vi "NI9252_AnalogInputWaveforms_v2.vi"() -> ()   [LabVIEW 2025]
uses:
  <vilib>/DAQmx/read.llb/DAQmx Read (Analog 1D Wfm NChan NSamp).vi
  <vilib>/DAQmx/configure/timing.llb/DAQmx Timing (Sample Clock).vi
  <vilib>/DAQmx/miscellaneous.llb/DAQmx Fill In Error Info.vi
panel:
  out "error out":errorcluster
  out "AI6 - Angle Sensor":dynamicdata(graph)
  out "AI5 - Potentiometer Sensor":dynamicdata(graph)
  out "AI4 - Differential Pressure":dynamicdata(graph)
  out "AI3 - Chamber Pressure":dynamicdata(graph)
  out "AI1 - Flow Meter Pressure":dynamicdata(graph)
  out "AI2 - Inlet Pressure":dynamicdata(graph)
  out "AI0 - Supply Pressure":dynamicdata(graph)
  in  "stop":bool
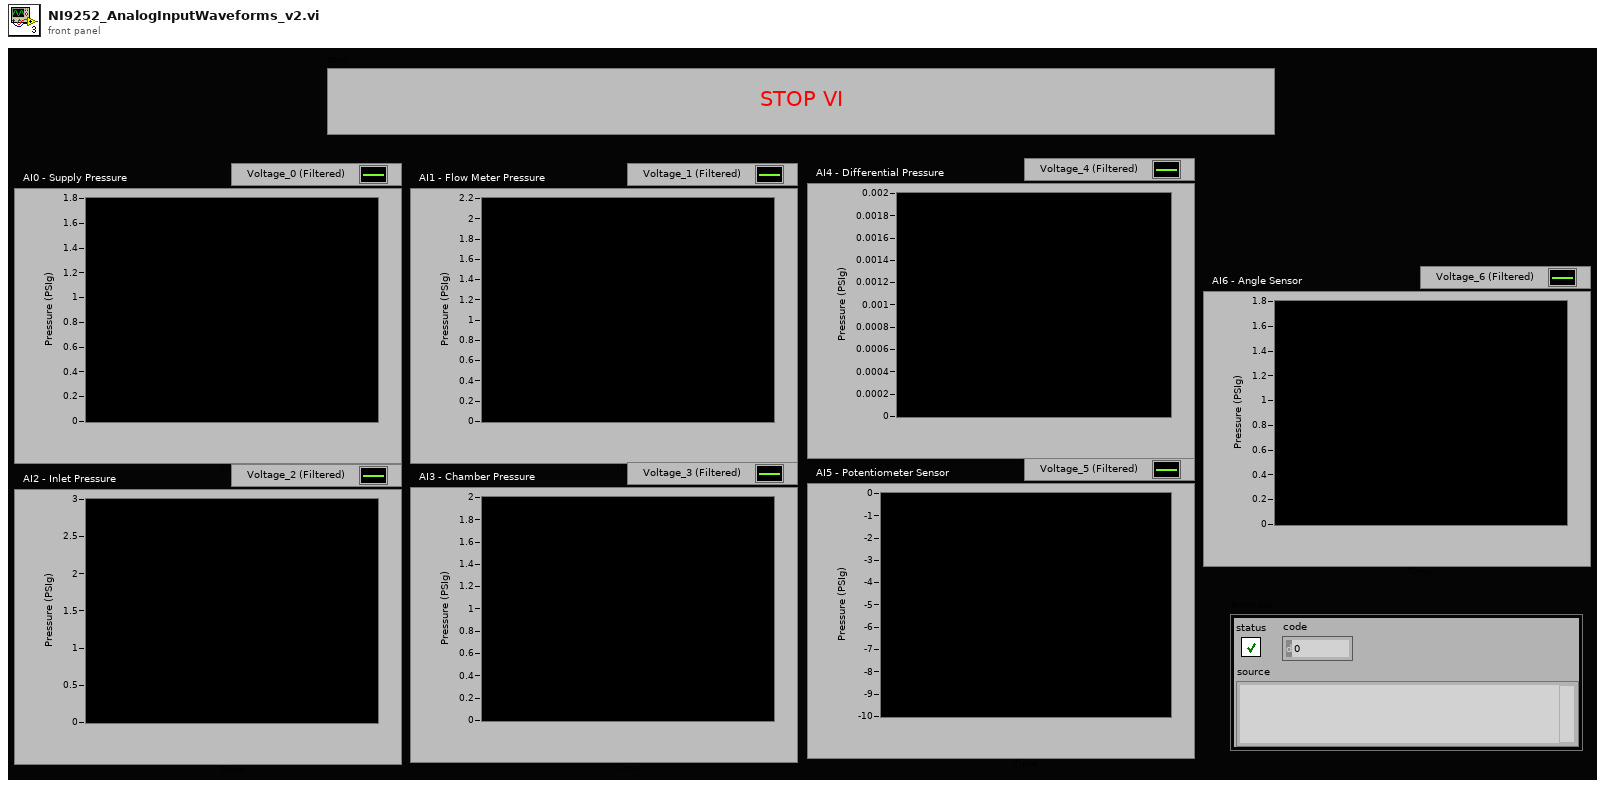
[diagram p1: front panel]
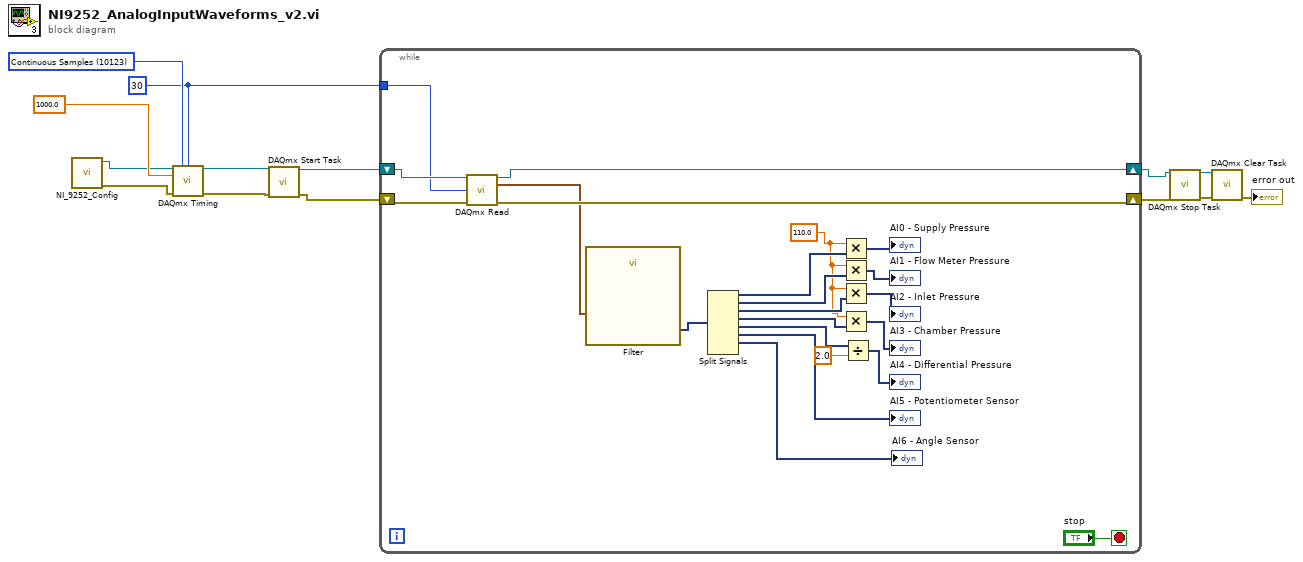
[diagram p0: block diagram]
diagram:
  w6 = 30 ("samples per channel")
  w7 = 10123 items=["Finite Samples"=10178, "Continuous Samples"=10123, "Hardware Timed Single Point"=12522] ("sample mode")
  n1 = call "NI_9252_Config.vi"() -> ("error out"=w12:errorcluster, "task out"=w13:refnum<k21>)  [unwired: 10 in]
  n2 = call-poly <vilib>:"DAQmx Timing.vi"("task/channels in"=w13, "sample mode"=w7, "samples per channel"=w6, "rate"=1000.0, "error in"=w12) -> ("task out"=w11:refnum<k21>, "error out"=w10:errorcluster)  [unwired: 9 in]
  n3 = call <vilib>:"DAQmx Start Task.vi"("task/channels in"=w11, "error in"=w10) -> ("task out"=w9:refnum<k21>, "error out"=w8:errorcluster)  [unwired: 12 in]
  n4 = while {
    shift-right: [w34] -> w4
    shift-left: w9 -> [w36]
    shift-right: [w33] -> w3
    shift-left: w8 -> [w15]
    tunnel: w6 -> [w35]
    stop <- "stop" stop-if-true
    w24 = 110.0
    n5 = call-poly <vilib>:"DAQmx Read.vi"("task/channels in"=w36, "number of samples per channel"=w35, "error in"=w15) -> ("task out"=w34:refnum<k21>, "data"=w23:waveform(dbl)[], "error out"=w33:errorcluster)  [unwired: 10 in]
    n6 = call "Filter"("Signal"=w23) -> ("Filtered Signal"=w22:dynamicdata)  [unwired: 9 in, 1 out]
    n7 = Split Signals(w22) -> (w31:dynamicdata, w30:dynamicdata, w29:dynamicdata, w28:dynamicdata, w20:dynamicdata, →"AI5 - Potentiometer Sensor":dynamicdata, →"AI6 - Angle Sensor":dynamicdata)  [unwired: 8 in, 1 out]
    n8 = Multiply(x=w24, y=w31) -> (x*y=→"AI0 - Supply Pressure":dynamicdata)
    n9 = Multiply(x=w24, y=w30) -> (x*y=→"AI1 - Flow Meter Pressure":dynamicdata)
    n10 = Multiply(x=w24, y=w29) -> (x*y=→"AI2 - Inlet Pressure":dynamicdata)
    n11 = Multiply(x=w24, y=w28) -> (x*y=→"AI3 - Chamber Pressure":dynamicdata)
    n12 = Divide(x=w20, y=2.0) -> (x/y=→"AI4 - Differential Pressure":dynamicdata)
  }
  n13 = call <vilib>:"DAQmx Stop Task.vi"("task/channels in"=w4, "error in"=w3) -> ("task out"=w1:refnum<k21>, "error out"=w5:errorcluster)  [unwired: 12 in]
  n14 = call <vilib>:"DAQmx Clear Task.vi"("task in"=w1, "error in"=w5) -> ("error out"=→"error out":errorcluster)  [unwired: 13 in]
